vi "ACIR.vi"(6 "Setting":T1={"Freq"=1000.0, "Range"=enum."10m Ohm", "Measurements"=enum."OCV"} {"Freq" min=0.1 max=1050.0 step=0.01 format="%_5e"}, 8 "error in":errorcluster, 9 "ACIR Ref":string, 10 "ACIR Class":string="Sim ACIR\\Sim ACIR.lvclass", 11 "Base Path":path=path "C:/GitHub/OOP Template/HAL/Concrete") -> (0 "error out":errorcluster, 3 "Measurements":dbl=6.933884571304798e-05)   [LabVIEW 2019, in "MAL.lvlib"]
uses:
  MAL.lvlib
  Hardware Abstraction/Harware Abstraction/Analog In/Analog In.lvclass
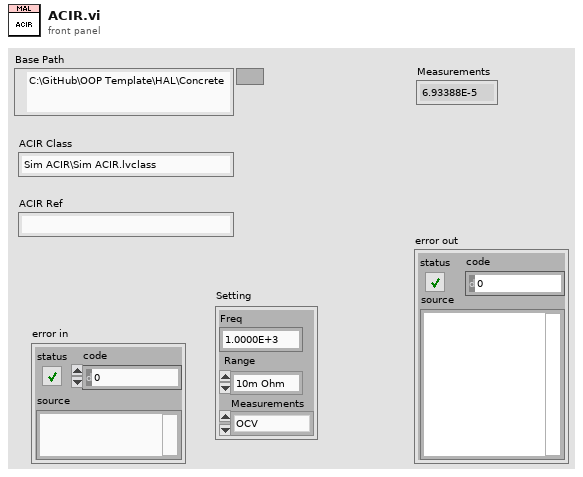
[diagram p1: front panel]
types:
  T1 = cluster{"Freq":dbl, "Range":enum16{"3m Ohm", "10m Ohm", "100m Ohm"}, "Measurements":enum16{"Impedence", "Phase Angle", "OCV"}}
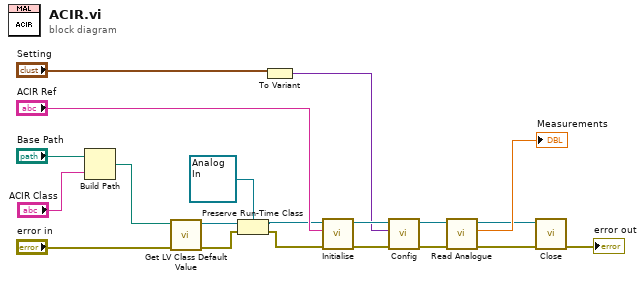
[diagram p0: block diagram]
diagram:
  n1 = Build Path(base path="Base Path", name or relative path="ACIR Class") -> (appended path=w14:path)
  n2 = call <vilib>:"Get LV Class Default Value.vi"("error in (no error)"="error in", "class path"=w14) -> ("error out"=w19:errorcluster, "object"=w20:refnum<class>)  [unwired: 8 in]
  n3 = Preserve Run-Time Class(object in=w20, error in=w19, 2:refnum<class "Analog In.lvclass"> refnum ("Hardware Abstration.lvlib:Analog In.lvclass")) -> (object out=w12:refnum<class "Analog In.lvclass">, error out=w17:errorcluster)
  n4 = To Variant(anything="Setting") -> (Variant=w1:variant)
  n5 = call-dynamic "Initialise.vi"("error in (no error)"=w17, "Instrument Ref"="ACIR Ref", "Instrument in"=w12) -> ("error out"=w4:errorcluster, "Instrument out"=w6:refnum<class "Analog In.lvclass">)  [unwired: 7 in]
  n6 = call-dynamic "Config.vi"("error in (no error)"=w4, "Setting"=w1, "Analog In in"=w6) -> ("error out"=w3:errorcluster, "Analog In out"=w5:refnum<class "Analog In.lvclass">)  [unwired: 7 in]
  n7 = call-dynamic "Read Analogue.vi"("error in (no error)"=w3, "PS in"=w5) -> ("error out"=w9:errorcluster, "Measurements"=→"Measurements":dbl, "PS out"=w7:refnum<class "Analog In.lvclass">)  [unwired: 7 in]
  n8 = call-dynamic "Close.vi"("error in (no error)"=w9, "Instrument in"=w7) -> ("error out"=→"error out":errorcluster)  [unwired: 8 in, 1 out]
